vi "Teleop.vi"(10 "Match Info":T1={"Autonomous Elapsed Seconds"=0.0, "TeleOp Elapsed Seconds"=0.0, "Disabled Elapsed Seconds"=0.0, "Visited Autonomous"=FALSE, "Visited TeleOp"=FALSE, "Visited Disabled"=FALSE, "Autonomous Settings"={"Autonomous Style"=enum."Independent", "VI Refnum"=refnum}}, 11 "Call Context":T2) -> ()   [LabVIEW 2017]
doc: "This VI is called for each TeleOp packet received from the DS where the robot is not disabled. It is often used to read from the joysticks and update I/O or to update setpoints for timed control loops. It should complete and return within 20 milliseconds or it may miss DS packets."
uses:
  <vilib>/Rock Robotics/WPI/DriverStation/WPI_DriverStationDerivedRobotMode.ctl
  <vilib>/Rock Robotics/WPI/DriverStation/WPI_DriverStationMatch Info.ctl
  <vilib>/Rock Robotics/WPI/ThirdParty/Phoenix-LabVIEW/Motor Controller/Controls/CTRE_Phoenix_MotorControl_ControlMode.ctl
  <vilib>/Rock Robotics/WPI/ThirdParty/Sensors/navX/_TypeDefs/Flags/Z900_navX_Flags_OpStatusTypeDef.ctl
  <vilib>/Rock Robotics/WPI/Utilities/WPI_GetSetVariantRefNum.vi
  <vilib>/Rock Robotics/Network Tables/NT Write Boolean Array.vi
  <vilib>/Rock Robotics/Network Tables/NT Write Numeric Array.vi
  <vilib>/Rock Robotics/Network Tables/NT Read Boolean.vi
  <vilib>/Rock Robotics/Network Tables/NT Read Number.vi
  <vilib>/Rock Robotics/WPI/ThirdParty/Phoenix-LabVIEW/Pigeon IMU/CTRE_PigeonIMU_GetTempStateUpTime.vi
  <vilib>/Rock Robotics/WPI/ThirdParty/Phoenix-LabVIEW/Pigeon IMU/CTRE_PigeonIMU_GetFusedHeading.vi
  <vilib>/Rock Robotics/WPI/ThirdParty/Phoenix-LabVIEW/Pigeon IMU/CTRE_PigeonIMU_GetYPR.vi
panel:
  in  "Self Righting":bool
  out "lift":dbl
  in  "D Gain":dbl=0.0004 format="%#_13g"
  in  "P Gain":dbl=0.04 format="%#_13g"
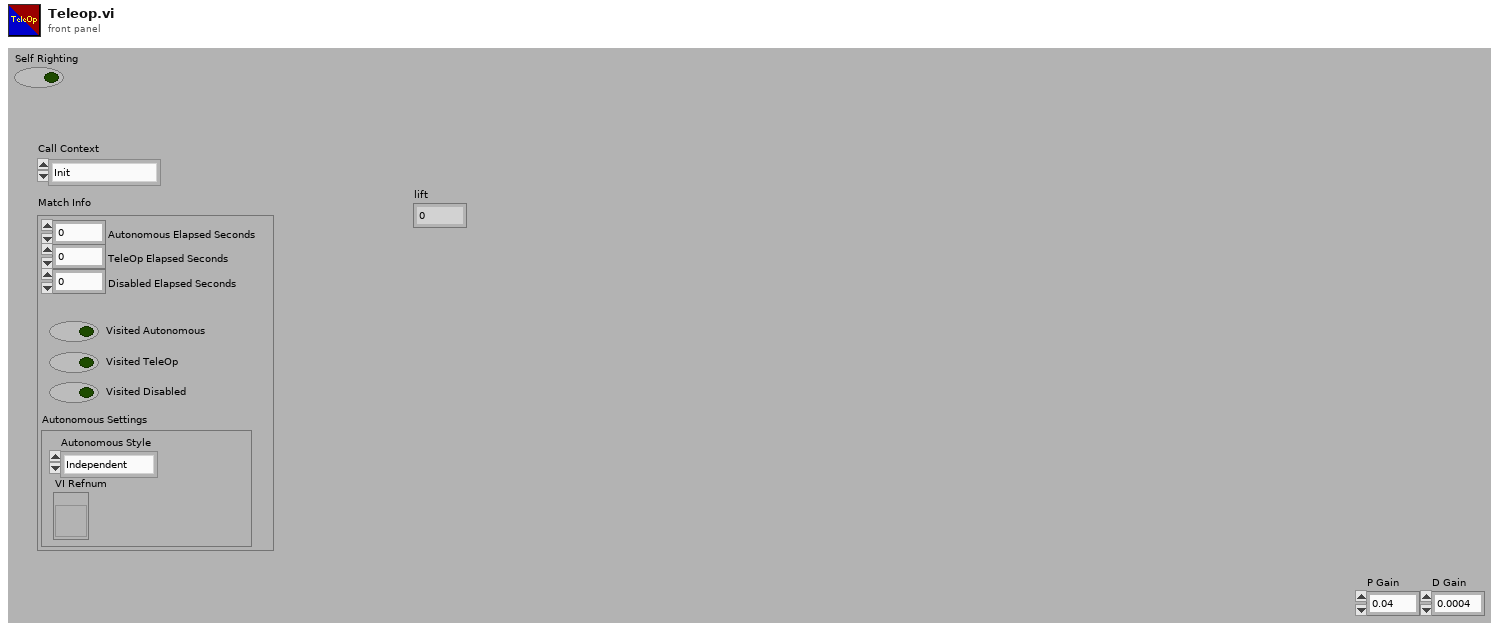
[diagram p1: front panel]
types:
  T1 = typedef "WPI_DriverStationMatch Info.ctl" = cluster{"Autonomous Elapsed Seconds":dbl, "TeleOp Elapsed Seconds":dbl, "Disabled Elapsed Seconds":dbl, "Visited Autonomous":bool, "Visited TeleOp":bool, "Visited Disabled":bool, "Autonomous Settings":cluster{"Autonomous Style":enum16{"Iterative", "Independent"}, "VI Refnum":refnum<vi>}}
  T2 = typedef "WPI_DriverStationDerivedRobotMode.ctl" = enum16{"Init", "Execute", "Stop"}
  T3 = typedef "CTRE_Phoenix_MotorControl_ControlMode.ctl" = u16
  T4 = typedef "WPI_JoystickDevRef.ctl" = cluster{"Device":T5}
  T5 = typedef "WPI_JoystickDeviceEnum.ctl" = enum16{"USB 0", "USB 1", "USB 2", "USB 3", "USB 4", "USB 5"}
  T6 = cluster{"Axes[0]":dbl, "Axes[1]":dbl, "Axes[2]":dbl, "Axes[3]":dbl, "Axes[4]":dbl, "Axes[5]":dbl, "Axes[6]":dbl, "Axes[7]":dbl, "Axes[8]":dbl}
  T7 = typedef "WPI_MotorControlDeviceRef.ctl" = cluster{"DeviceStatus":errorcluster, "Type":T8, "PWM":cluster{"PWM Channel":T9, "DeadBand":T10}, "CAN":cluster{"Device Number":u8, "SetOutput VI Ref":variant, "GetOutput VI Ref":variant, "Enable VI Ref":variant, "Disable VI Ref":variant, "Data":variant}, "Invert":bool, "DIO PWM":cluster{"PWM \"Enable\" Channel":T9, "DIOChannel":T11, "PWM Rate":dbl}}
  T8 = typedef "WPI_MotorControlType.ctl" = enum16{"PWM", "CAN", "DIO PWM"}
  T9 = typedef "FPGA_DIOPWMChannel.ctl" = enum8{"PWM 0", "PWM 1", "PWM 2", "PWM 3", "PWM 4", "PWM 5", "PWM 6", "PWM 7", "PWM 8", "PWM 9", "PWM MXP 0", "PWM MXP 1", "PWM MXP 2", "PWM MXP 3", "PWM MXP 4", "PWM MXP 5", "PWM MXP 6", "PWM MXP 7", "PWM MXP 8", "PWM MXP 9", "Invalid"}
  T10 = typedef "WPI_PWMDeadband.ctl" = cluster{"Name":string, "maxPositivePwm":i32, "minPositivePwm":i32, "centerPwm":i32, "maxNegativePwm":i32, "minNegativePwm":i32, "angularRange":u16}
  T11 = typedef "FPGA_DIOChannel.ctl" = enum8{"DIO 0", "DIO 1", "DIO 2", "DIO 3", "DIO 4", "DIO 5", "DIO 6", "DIO 7", "DIO 8", "DIO 9", "DIO MXP 0", "DIO MXP 1", "DIO MXP 2", "DIO MXP 3", "DIO MXP 4", "DIO MXP 5", "DIO MXP 6", "DIO MXP 7", "DIO MXP 8", "DIO MXP 9", "DIO MXP 10", "DIO MXP 11", "DIO MXP 12", "DIO MXP 13", "DIO MXP 14", "DIO MXP 15", "SPI Port CS1", "SPI Port CS2", "SPI Port CS3", "SPI Port MISO", "SPI Port MOSI", "Invalid"}
  T12 = typedef "CTRE_PigeonIMU_DeviceRef.ctl" = cluster{"DeviceStatus":errorcluster, "Device Number":u8, "Type":T13, "Device ID":u32, "Handle":u64, "UsageFrame":u32, "Library Path":path}
  T13 = typedef "CTRE_PigeonIMU_ConnectionType.ctl" = u32
  T14 = typedef "CTRE_PigeonIMU_CalibrationMode.ctl" = u16
  T15 = typedef "CTRE_PigeonIMU_PigeonState.ctl" = enum16{"NoComm", "Initializing", "Ready", "UserCalibration"}
  T16 = cluster{"CurrentMode":T14, "LastCalError":i32, "CalBooting?":bool, "PigeonState":T15, "UpTime":u32, "Temp. (C)":dbl, "Temp Compensation Event Count":u32, "No Motion Event Count":u32}
  T17 = cluster{"Heading":dbl, "Valid?":bool, "Fusing?":bool}
  T18 = typedef "Z900_navX_Flags_OpStatusTypeDef.ctl" = u8
  T19 = typedef "WPI_RobotDriveDevRef.ctl" = cluster{"DevStatus":errorcluster, "Motors[]":T7[], "Square Inputs":bool, "Max Output":dbl}
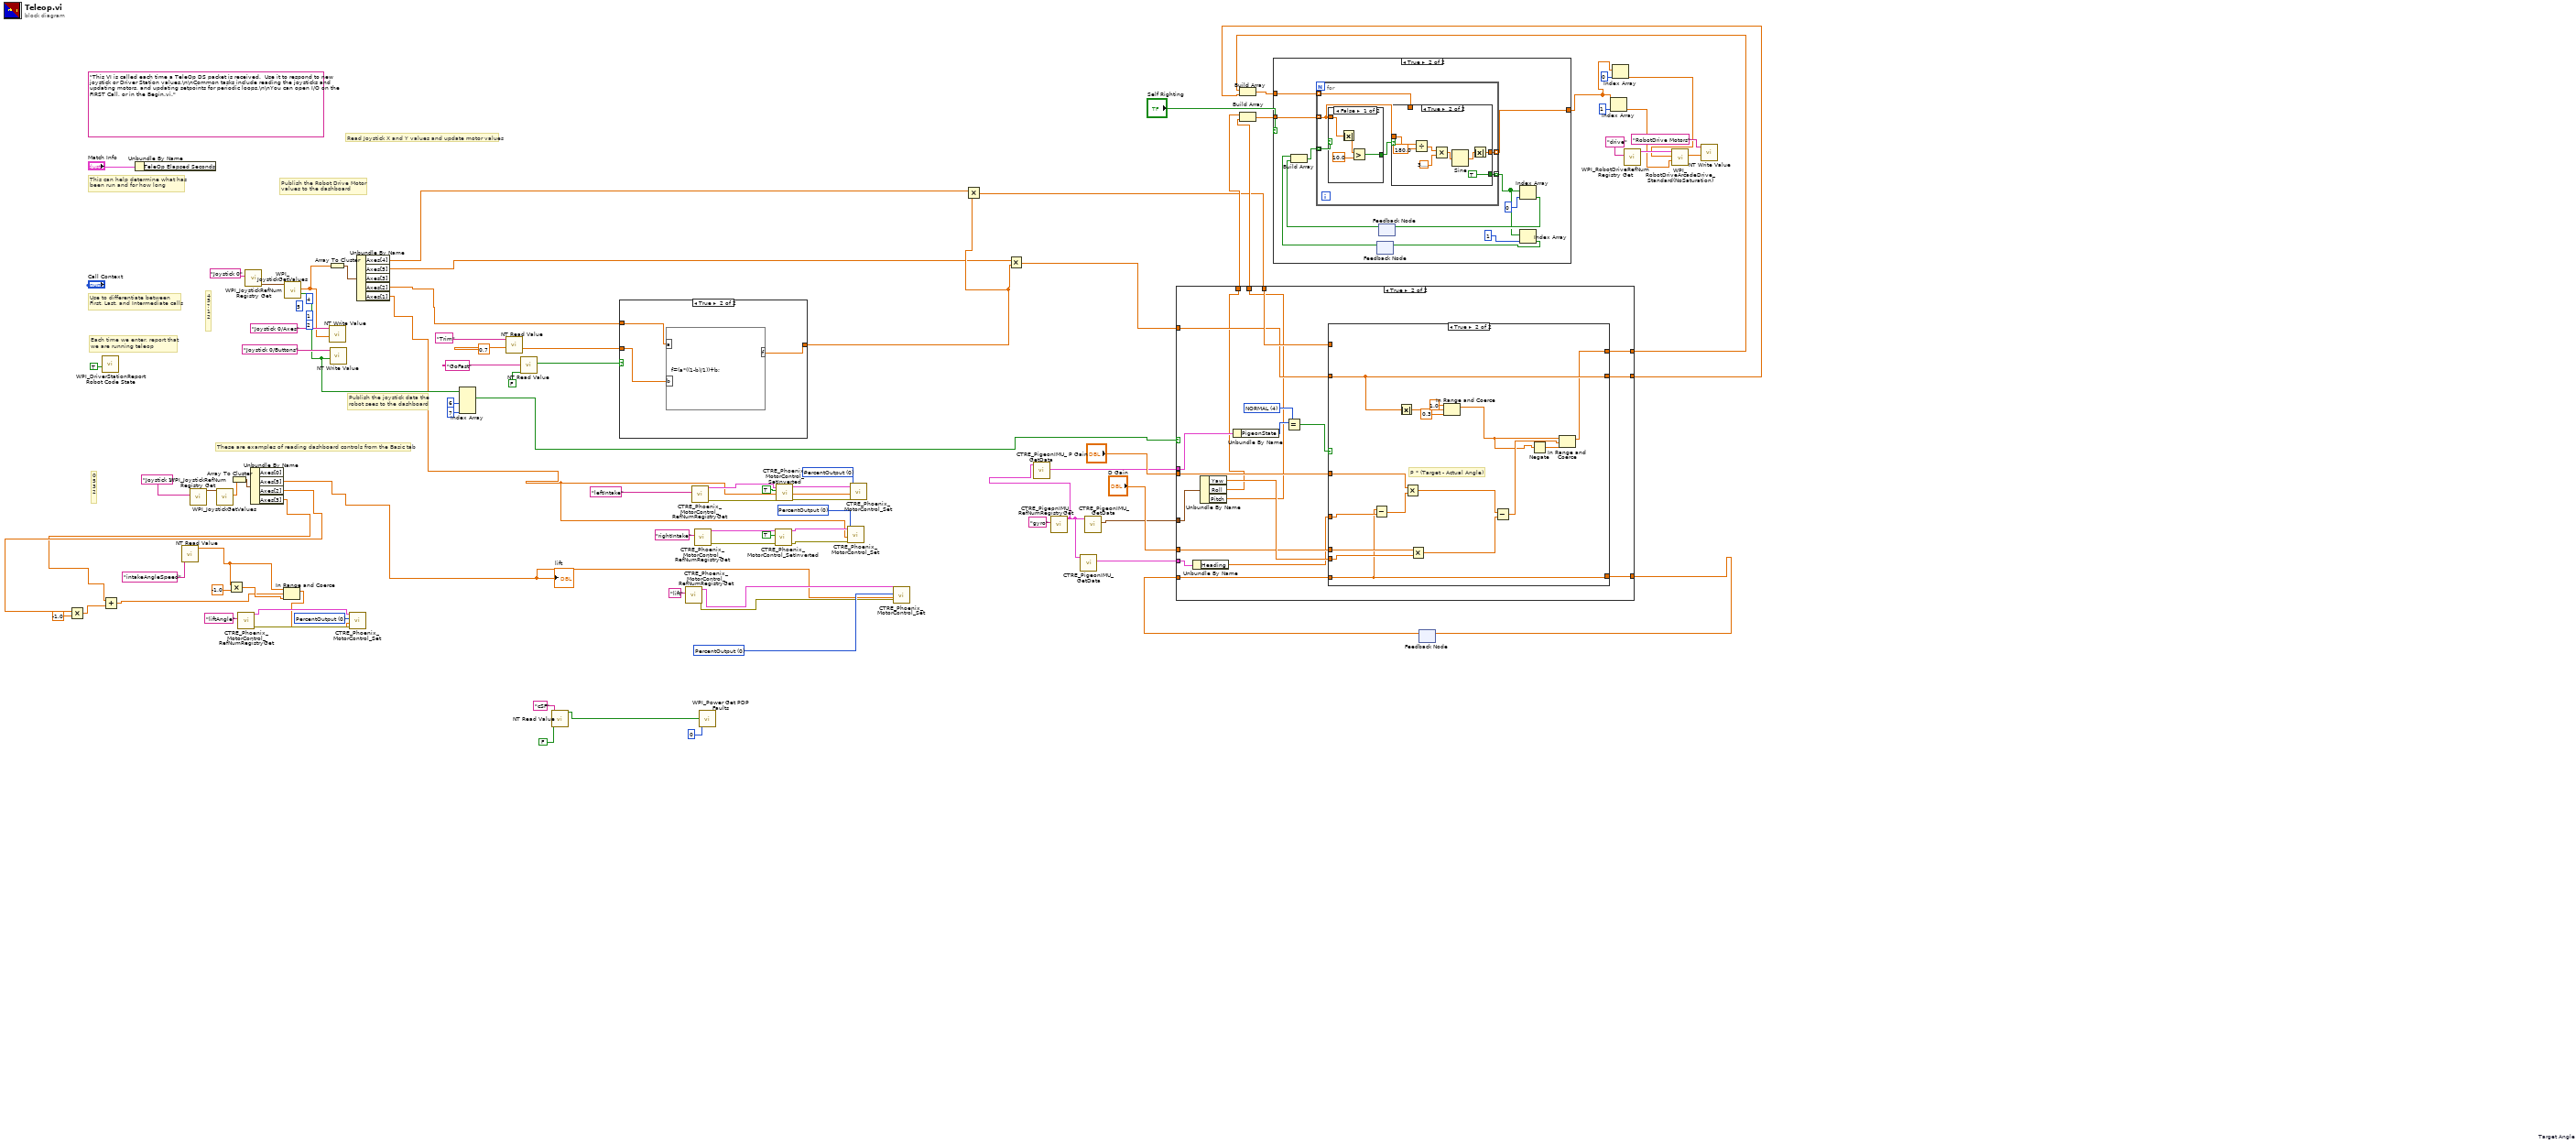
[diagram p0: block diagram]
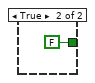
[diagram p4: hidden frame]
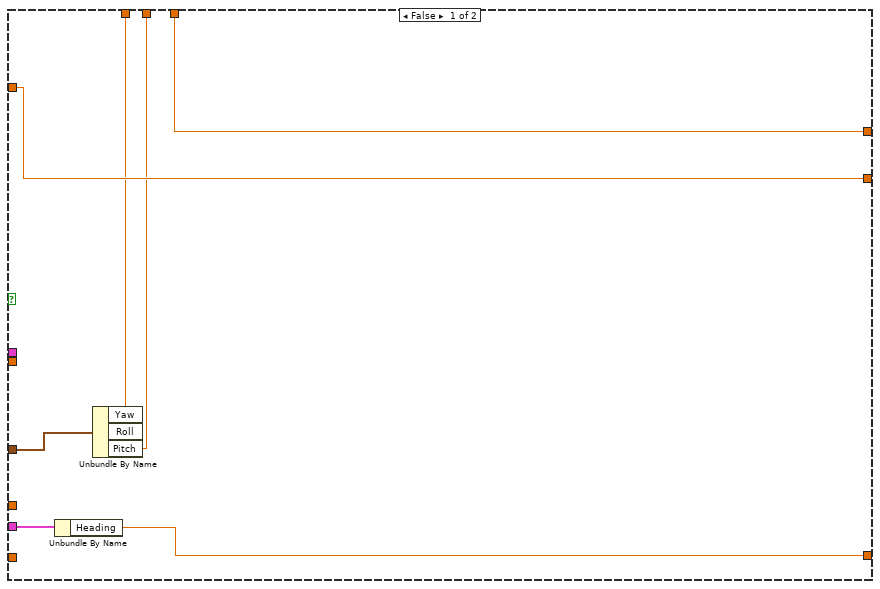
[diagram p5: hidden frame]
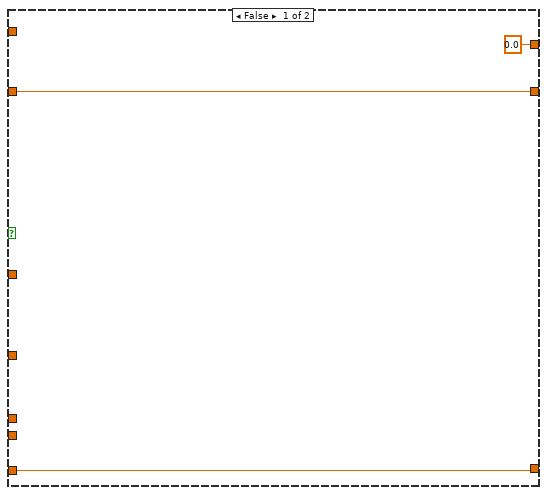
[diagram p6: hidden frame]
diagram:
  (unwired) 2 ("index")
  (unwired) 5 ("index")
  (unwired) 4 ("index")
  w43 = T3 0 items=["PercentOutput"=0, "Position"=1, "Velocity"=2, "Current"=3, "Follower"=5, "MotionProfile"=6, "MotionMagic"=7, "MotionMagicArc"=8, "MotionProfileArc"=10, "Disabled"=15] ("Control Mode")
  (unwired) 1 ("index")
  w44 = T3 0 items=["PercentOutput"=0, "Position"=1, "Velocity"=2, "Current"=3, "Follower"=5, "MotionProfile"=6, "MotionMagic"=7, "MotionMagicArc"=8, "MotionProfileArc"=10, "Disabled"=15] ("Control Mode")
  w45 = T3 0 items=["PercentOutput"=0, "Position"=1, "Velocity"=2, "Current"=3, "Follower"=5, "MotionProfile"=6, "MotionMagic"=7, "MotionMagicArc"=8, "MotionProfileArc"=10, "Disabled"=15] ("Control Mode")
  w52 = T3 0 items=["PercentOutput"=0, "Position"=1, "Velocity"=2, "Current"=3, "Follower"=5, "MotionProfile"=6, "MotionMagic"=7, "MotionMagicArc"=8, "MotionProfileArc"=10, "Disabled"=15] ("Control Mode")
  (unwired) "This VI is called each time a TeleOp DS packet is received.  Use it to respond to new joystick or Driver Station values.\n\nCommon tasks include reading the joysticks and updating motors, and updating setpoints for periodic loops.\n\nYou can open I/O on the FIRST Call, or in the Begin.vi."
  # "4\n5\n?\n1\n2"
  # "0\n5\n3\n2"
  # "These are examples of reading dashboard controls from the Basic tab"
  # "Publish the Robot Drive Motor\nvalues to the dashboard"
  # "Publish the joystick data the\nrobot sees to the dashboard"
  # "Each time we enter, report that\nwe are running teleop"
  # "Use to differentiate between\nFirst, Last, and Intermediate calls"
  # "This can help determine what has\nbeen run and for how long"
  # "Read Joystick X and Y values and update motor values"
  n1 = call <vilib>:"WPI_DriverStationReport Robot Code State.vi"("TeleOp"=TRUE ("Autonomous")) -> ()  [unwired: 10 in, 1 out]
  n2 = Unbundle By Name("Match Info") -> ()  [unwired: 1 out]
  n3 = call-poly <vilib>:"NT Read Value.vi"("Name"="intakeAngleSpeed") -> ("Numeric"=w37:dbl)  [unwired: 9 in, 1 out]
  n4 = call <vilib>:"WPI_JoystickRefNum Registry Get.vi"("refnum name"="Joystick 1") -> ("JoystickDevRef"=w48:T4)  [unwired: 1 in, 9 out]
  n5 = call <vilib>:"WPI_JoystickGetValues.vi"("JoystickDevRef"=w48) -> ("Axes"=w11:dbl[])  [unwired: 6 in, 4 out]
  n6 = Multiply(x=w37, y=-1.0) -> (x*y=w35:dbl)
  n7 = Array To Cluster(array=w11) -> (cluster=w10:T6)
  n8 = call <vilib>:"CTRE_Phoenix_MotorControl_RefNumRegistryGet.vi"("refnum name"="liftAngle") -> ("error out"=w40:errorcluster, "PhoenixMotorControlDevRef"=w41:T7)  [unwired: 9 in]
  n9 = call <vilib>:"WPI_JoystickRefNum Registry Get.vi"("refnum name"="Joystick 0") -> ("JoystickDevRef"=w87:T4)  [unwired: 1 in, 9 out]
  n10 = Unbundle By Name(w10) -> ("Axes[5]"=w9:dbl, "Axes[2]"=w8:dbl, "Axes[3]"=w7:dbl)  [unwired: 1 out]
  "lift" <- w9
  n11 = Multiply(x=w8, y=-1.0) -> (x*y=w18:dbl)
  n12 = Add(x=w7, y=w18) -> (x+y=w17:dbl)
  n13 = In Range and Coerce(upper limit=w37, x=w17, lower limit=w35) -> (coerced(x)=w39:dbl)  [unwired: 1 out]
  n14 = call <vilib>:"WPI_JoystickGetValues.vi"("JoystickDevRef"=w87) -> ("Buttons"=w70:bool[], "Axes"=w6:dbl[])  [unwired: 6 in, 3 out]
  n15 = Array To Cluster(array=w6) -> (cluster=w5:T6)
  n16 = call-poly <vilib>:"NT Write Value.vi"("Numeric Array"=w6, "Name"="Joystick 0/Axes") -> ()  [unwired: 9 in, 1 out]
  n17 = call-poly <vilib>:"NT Write Value.vi"("Boolean Array"=w70, "Name"="Joystick 0/Buttons") -> ()  [unwired: 9 in, 1 out]
  n18 = call <vilib>:"CTRE_Phoenix_MotorControl_Set.vi"("error in (no error)"=w40, "Output"=w39, "Control Mode"=w43, "PhoenixMotorControlDevRef"=w41) -> ()  [unwired: 6 in, 2 out]
  n19 = Unbundle By Name(w5) -> ("Axes[4]"=w4:dbl, "Axes[5]"=w3:dbl, "Axes[2]"=w1:dbl, "Axes[1]"=w2:dbl)  [unwired: 1 out]
  n20 = Index Array(array=w70, index #2=6 ("index"), index #3=7 ("index")) -> (element #1=w69:bool)  [unwired: 2 in, 3 out]
  n21 = call-poly <vilib>:"NT Read Value.vi"("Default Value"=0.7, "Name"="Trim" ("refnum name")) -> ("Numeric"=w76:dbl)  [unwired: 8 in, 1 out]
  n22 = call-poly <vilib>:"NT Read Value.vi"("Default Value"=FALSE, "Name"="GoFast" ("refnum name")) -> ("Boolean"=w77:bool)  [unwired: 8 in, 1 out]
  n23 = call-poly <vilib>:"NT Read Value.vi"("Default Value"=FALSE, "Name"="cSF") -> ("Boolean"=w32:bool)  [unwired: 8 in, 1 out]
  n24 = case shown="True" w77 {
    tunnel: [w92 w95] -> w75
    tunnel: w76 -> [w92 w94]
    tunnel: w1 -> [_ w93]
    frame False {
    }
    frame True {
      n25 = formula code="f=(a*((1-b)/1))+b;"("a"=w93, "b"=w94) -> ("f"=w95:dbl)
    }
  }
  n26 = call <vilib>:"CTRE_Phoenix_MotorControl_RefNumRegistryGet.vi"("refnum name"="lift") -> ("error out"=w34:errorcluster, "PhoenixMotorControlDevRef"=w33:T7)  [unwired: 9 in]
  n27 = call <vilib>:"CTRE_Phoenix_MotorControl_RefNumRegistryGet.vi"("refnum name"="leftIntake") -> ("error out"=w27:errorcluster, "PhoenixMotorControlDevRef"=w28:T7)  [unwired: 9 in]
  n28 = call <vilib>:"CTRE_Phoenix_MotorControl_RefNumRegistryGet.vi"("refnum name"="rightIntake") -> ("error out"=w23:errorcluster, "PhoenixMotorControlDevRef"=w24:T7)  [unwired: 9 in]
  n29 = call <vilib>:"WPI_Power Get PDP Faults.vi"("Power Distribution Panel (0)"=u8 0, "Clear Sticky Faults"=w32) -> ()  [unwired: 9 in, 5 out]
  n30 = call <vilib>:"CTRE_Phoenix_MotorControl_SetInverted.vi"("error in (no error)"=w23, "Invert?"=TRUE, "PhoenixMotorControlDevRef"=w24) -> ("error out"=w21:errorcluster, "PhoenixMotorControlDevRef"=w22:T7)  [unwired: 7 in]
  n31 = call <vilib>:"CTRE_Phoenix_MotorControl_SetInverted.vi"("error in (no error)"=w27, "Invert?"=TRUE, "PhoenixMotorControlDevRef"=w28) -> ("error out"=w25:errorcluster, "PhoenixMotorControlDevRef"=w26:T7)  [unwired: 7 in]
  n32 = call <vilib>:"CTRE_Phoenix_MotorControl_Set.vi"("error in (no error)"=w21, "Output"=w2, "Control Mode"=w45, "PhoenixMotorControlDevRef"=w22) -> ()  [unwired: 6 in, 2 out]
  n33 = call <vilib>:"CTRE_Phoenix_MotorControl_Set.vi"("error in (no error)"=w25, "Output"=w2, "Control Mode"=w44, "PhoenixMotorControlDevRef"=w26) -> ()  [unwired: 6 in, 2 out]
  n34 = call <vilib>:"CTRE_Phoenix_MotorControl_Set.vi"("error in (no error)"=w34, "Output"=w9, "Control Mode"=w52, "PhoenixMotorControlDevRef"=w33) -> ()  [unwired: 6 in, 2 out]
  n35 = Multiply(x=w4, y=w75) -> (x*y=w57:dbl)
  n36 = Multiply(x=w3, y=w75) -> (x*y=w61:dbl)
  n37 = call <vilib>:"CTRE_PigeonIMU_RefNumRegistryGet.vi"("refnum name"="gyro") -> ("PigeonIMUDevRef"=w12:T12)  [unwired: 9 in, 1 out]
  n38 = call-poly <vilib>:"CTRE_PigeonIMU_GetData.vi"("PigeonIMUDevRef"=w12) -> ("Temp/State/UpTime"=w13:T16)  [unwired: 8 in, 2 out]
  n39 = call-poly <vilib>:"CTRE_PigeonIMU_GetData.vi"("PigeonIMUDevRef"=w12) -> ("Fused Heading"=w14:T17)  [unwired: 8 in, 2 out]
  n40 = call-poly <vilib>:"CTRE_PigeonIMU_GetData.vi"("PigeonIMUDevRef"=w12) -> ("Yaw Pitch Roll"=w15:cluster{"Yaw":dbl, "Pitch":dbl, "Roll":dbl})  [unwired: 8 in, 2 out]
  n41 = feedback #1 "Target Angle"() -> (w72:dbl)  [unwired: 1 in]
  n42 = case shown="True" w69 {
    tunnel: "P Gain" -> [_ w117]
    tunnel: "D Gain" -> [_ w116]
    tunnel: w72 -> [_ w115]
    tunnel: w57 -> [w102 w114]
    tunnel: w61 -> [w101 w113]
    tunnel: [w101 w112] -> w55
    tunnel: [w102 w111] -> w56
    tunnel: [w96 w110] -> w71
    tunnel: [w100 w103] -> w60
    tunnel: [w99 w104] -> w59
    tunnel: w15 -> [w98 w107]
    tunnel: w14 -> [w97 w106]
    tunnel: w13 -> [_ w109]
    frame False {
      n43 = Unbundle By Name(w97) -> ("Heading"=w96:dbl)
      n44 = Unbundle By Name(w98) -> ("Roll"=w100:dbl, "Pitch"=w99:dbl)  [unwired: 1 out]
    }
    frame True {
      w120 = T18 4 items=["INITIALIZING", "SELFTEST_IN_PROGRESS", "ERROR", "IMU_AUTOCAL_IN_PROGRESS", "NORMAL"] ("y")
      n45 = Unbundle By Name(w106) -> ("Heading"=w105:dbl)
      n46 = Unbundle By Name(w107) -> ("Yaw"=w118:dbl, "Roll"=w103:dbl, "Pitch"=w104:dbl)
      n47 = Unbundle By Name(w109) -> ("PigeonState"=w108:T15)
      n48 = Equal?(x=w108, y=w120) -> (x = y?=w119:bool)
      n49 = case shown="True" w119 {
        tunnel: w105 -> [_ w139]
        tunnel: w118 -> [_ w136]
        tunnel: w117 -> [_ w137]
        tunnel: w116 -> [_ w135]
        tunnel: w115 -> [w123 w124]
        tunnel: w114 -> [_ _]
        tunnel: w113 -> [w122 w132]
        tunnel: [w122 w132] -> w112
        tunnel: [0.0 ("upper limit") w125] -> w111
        tunnel: [w123 w124] -> w110
        frame False {
        }
        frame True {
          # "P * (Target - Actual Angle)"
          n50 = Subtract(x=w124, y=w139) -> (x-y=w138:dbl)
          n51 = Absolute Value(x=w132) -> (abs(x)=w131:dbl)
          n52 = Multiply(x=w137, y=w138) -> (x*y=w134:dbl)
          n53 = Multiply(x=w135, y=w136) -> (x*y=w133:dbl)
          n54 = In Range and Coerce(upper limit=1.0, x=w131, lower limit=0.3) -> (coerced(x)=w126:dbl)  [unwired: 1 out]
          n55 = Subtract(x=w134, y=w133) -> (x-y=w128:dbl)
          n56 = Negate(x=w126) -> (-x=w127:dbl)
          n57 = In Range and Coerce(upper limit=w126, x=w128, lower limit=w127) -> (coerced(x)=w125:dbl)  [unwired: 1 out]
        }
      }
    }
  }
  n58 = Build Array(w56, w55) -> (w62:dbl[])
  n59 = Build Array(w60, w59) -> (w58:dbl[])
  n60 = case shown="True" "Self Righting" {
    tunnel: [w140 w151] -> w63
    tunnel: w62 -> [w140 w150]
    tunnel: w58 -> [_ w149]
    frame False {
    }
    frame True {
      n61 = feedback #2() -> (w144:bool)  [unwired: 1 in]
      n62 = feedback #3() -> (w145:bool)  [unwired: 1 in]
      n63 = Build Array(w144, w145) -> (w146:bool[])
      n64 = for {
        tunnel: [w157] -> w151 mode=indexing
        tunnel: w150 -> [w156] mode=indexing
        tunnel: w149 -> [w155] mode=indexing
        tunnel: [w154] -> w141 mode=indexing
        tunnel: w146 -> [w152] mode=indexing
        n65 = case shown="False" w152 {
          tunnel: w155 -> [w170 _]
          tunnel: [w168 FALSE] -> w153
          frame False {
            n66 = Absolute Value(x=w170) -> (abs(x)=w171:dbl)
            n67 = Greater?(x=w171, y=10.0) -> (0:w168:bool)
          }
          frame True {
          }
        }
        n68 = case shown="True" w153 {
          selector: w153 -> [w158 _]
          tunnel: [w159 w164] -> w157
          tunnel: w156 -> [w159 _]
          tunnel: w155 -> [_ w163]
          tunnel: [w158 TRUE] -> w154
          frame False {
          }
          frame True {
            n69 = Divide(x=w163, y=180.0) -> (x/y=w167:dbl)
            n70 = Multiply(x=w167, y=3.141592653589793) -> (x*y=w166:dbl)
            n71 = Sine(x=w166) -> (sin(x)=w165:dbl)
            n72 = Absolute Value(x=w165) -> (abs(x)=w164:dbl)
          }
        }
      }
      n73 = Index Array(array=w141, index=1) -> (element=w143:bool)
      n74 = feedback-in #2(w143) -> ()
      n75 = Index Array(array=w141, index=0) -> (element=w142:bool)
      n76 = feedback-in #3(w142) -> ()
    }
  }
  n77 = feedback-in #1(w71) -> ()
  n78 = Index Array(array=w63, index=1) -> (element=w54:dbl)
  n79 = Index Array(array=w63, index=0) -> (element=w53:dbl)
  n80 = call <vilib>:"WPI_RobotDriveRefNum Registry Get.vi"("refnum name"="drive") -> ("RobotDriveDevRef"=w89:T19)  [unwired: 1 in, 9 out]
  n81 = call <vilib>:"WPI_RobotDriveArcadeDrive_Standard(NoSaturation).vi"("Y axis value"=w54, "X axis value"=w53, "RobotDriveDevRef"=w89) -> ("Motor Values"=w83:dbl[])  [unwired: 1 in, 7 out]
  n82 = call-poly <vilib>:"NT Write Value.vi"("Numeric Array"=w83, "Name"="RobotDrive Motors") -> ()  [unwired: 9 in, 1 out]
